vi "Start Jl Server, Init LV client, check comm.vi"(0 "endpoint":string, 1 "delay after starting Julia":u32=3000, 5 "Julia ZMQ server file name":string, 9 "request":string, 11 "error in (no error)":errorcluster) -> (2 "LV client state":T1, 3 "JL server state":T1, 4 "zmq_context out":refnum<class "zmq_context.lvclass">, 6 "zmq_socket out":refnum<class "zmq_socket.lvclass">, 8 "response":string, 10 "return code":i32, 15 "error out":errorcluster)   [LabVIEW 2018, in "LV-Julia_ZMQ-Roundtrip_lib.lvlib"]
uses:
  LV-Julia_ZMQ-Roundtrip_lib.lvlib
  Server or client state.ctl
  <vilib>/addons/zeromq/zmq_socket.lvclass
  <vilib>/addons/zeromq/zmq_context.lvclass
  fd3403e4-487e-45c1-aab1-3d240bb50c66.vi
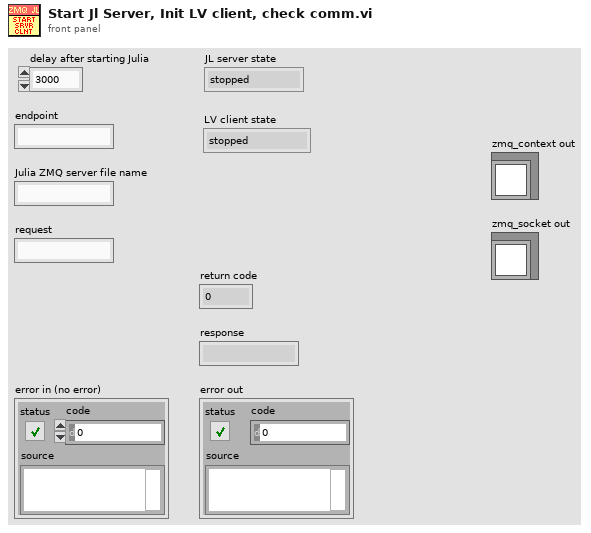
[diagram p1: front panel]
types:
  T1 = typedef "LV-Julia_ZMQ-Roundtrip_lib.lvlib/Server or client state.ctl" = enum16{"stopped", "running", "unknown"}
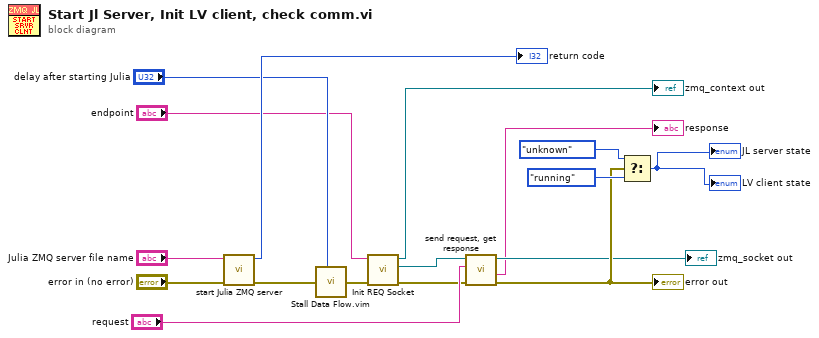
[diagram p0: block diagram]
diagram:
  n1 = call "start Julia ZMQ server.vi"("error in (no error)"="error in (no error)", "Julia ZMQ server file name"="Julia ZMQ server file name") -> ("error out"=w11:errorcluster, "return code"=→"return code":i32)  [unwired: 8 in]
  n2 = call "Stall Data Flow.vim"("value in"=w11, "milliseconds to wait"="delay after starting Julia") -> ("value out"=w14:errorcluster)  [unwired: 1 out]
  n3 = call "Init REQ Socket.vi"("error in (no error)"=w14, "endpoint"="endpoint") -> ("error out"=w3:errorcluster, "socket out"=w6:refnum<class "zmq_socket.lvclass">, "zmq_context out"=→"zmq_context out":refnum<class "zmq_context.lvclass">)  [unwired: 7 in]
  n4 = call "send request, get response.vi"("error in (no error)"=w3, "request"="request", "zmq_socket in"=w6) -> ("error out"=w9:errorcluster, "response"=→"response":string, "zmq_socket out"=→"zmq_socket out":refnum<class "zmq_socket.lvclass">)  [unwired: 4 in, 2 out]
  "error out" <- w9
  n5 = Select(t=Server_or_client_state."unknown" ("Server state"), s=w9, f=Server_or_client_state."running") -> (s? t:f=→"JL server state" →"LV client state":T1)
